vi "Date Name.vi"() -> (2 "Date Name":string)   [LabVIEW 2014, in "AvaSpec.lvlib" / "AvaSpec Logging.lvlib"]
uses:
  AvaSpec Logging.lvlib
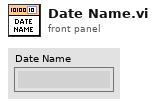
[diagram p1: front panel]
types:
  T1 = typedef "LVDateTimeRec.ctl" = cluster{"fractional second":dbl, "second":i32, "minute":i32, "hour":i32, "day of month":i32, "month":i32, "year":i32, "day of week":i32, "day of year":i32, "DST":i32}
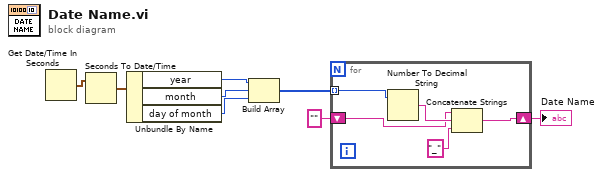
[diagram p0: block diagram]
diagram:
  n1 = Get Date/Time In Seconds() -> (seconds since 1Jan1904=w7:timestamp)
  n2 = Seconds To Date/Time(time stamp (now)=w7) -> (date time rec=w8:T1)  [unwired: 1 in]
  n3 = Unbundle By Name(w8) -> ("year"=w6:i32, "month"=w5:i32, "day of month"=w4:i32)
  n4 = Build Array(w6, w5, w4) -> (w3:i32[])
  n5 = for {
    tunnel: w3 -> [w13] mode=indexing
    shift-right: [w9] -> w1
    shift-left: "" -> [w11]
    n6 = Number To Decimal String(number=w13) -> (decimal integer string=w12:string)  [unwired: 1 in]
    n7 = Concatenate Strings(w11, w12, "_" ("element")) -> (w9:string)
  }
  "Date Name" <- w1
